vi "findBasePath.vi"(4 "path.in":path) -> (1 "path.out":path)   [LabVIEW 2015]
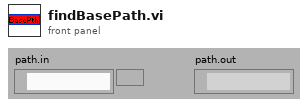
[diagram p1: front panel]
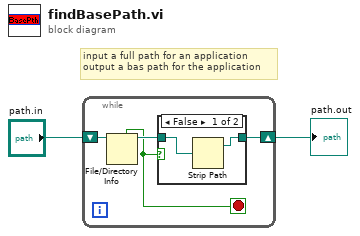
[diagram p0: block diagram]
diagram:
  # "input a full path for an application\noutput a bas path for the application"
  n1 = while {
    shift-right: [w4] -> w2
    shift-left: "path.in" -> [w6]
    stop <- w3 stop-if-true
    n2 = File/Directory Info(path=w6) -> (path out=w5:path, directory=w3:bool)  [unwired: 1 in, 5 out]
    n3 = case shown="False" w3 {
      tunnel: [w8 w9] -> w4
      tunnel: w5 -> [w7 w9]
      frame False {
        n4 = Strip Path(path=w7) -> (stripped path=w8:path)  [unwired: 1 out]
      }
      frame True {
      }
    }
  }
  "path.out" <- w2
